vi "No_of_steps.vi"(1 "Current position":i32, 2 "Desired position":i32) -> (0 "No of steps":i32)   [LabVIEW 2010]
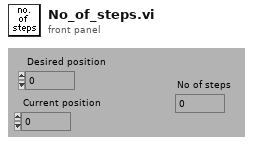
[diagram p1: front panel]
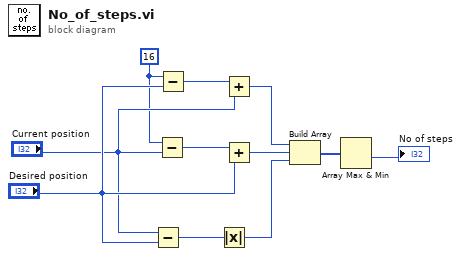
[diagram p0: block diagram]
diagram:
  w1 = 16
  n1 = Subtract(x="Current position", y="Desired position") -> (x-y=w10:i32)
  n2 = Subtract(x=w1, y="Current position") -> (x-y=w11:i32)
  n3 = Subtract(x=w1, y="Desired position") -> (x-y=w7:i32)
  n4 = Absolute Value(x=w10) -> (abs(x)=w4:i32)
  n5 = Add(x=w7, y="Current position") -> (x+y=w6:i32)
  n6 = Add(x=w11, y="Desired position") -> (x+y=w5:i32)
  n7 = Build Array(w6, w5, w4) -> (w3:i32[])
  n8 = Array Max & Min(array=w3) -> (min value=→"No of steps":i32)  [unwired: 3 out]
